vi "STOP.vi"(8 "error in (no error)":errorcluster, 11 "Stop in":refnum<class "DLEmulate.lvclass">) -> (0 "error out":errorcluster, 3 "Stop out":refnum<class "DLEmulate.lvclass">)   [LabVIEW 2015, in "DLEmulate.lvclass"]
uses:
  DLEmulate.lvclass
  GeneralFunctionality/GeneralFunctionality.lvclass/GeneralFunctionality.ctl
  GeneralFunctionality/GeneralFunctionality.lvclass
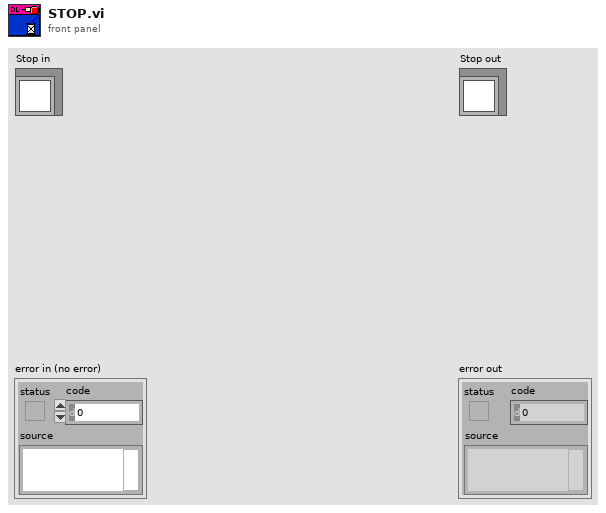
[diagram p1: front panel]
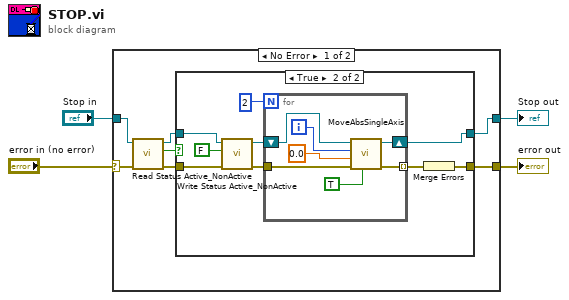
[diagram p0: block diagram]
diagram:
  n1 = case shown="No Error" "error in (no error)" {
    selector: "error in (no error)" -> [w8 w31]
    tunnel: [w11 w31] -> w2
    tunnel: [w5 w30] -> w1
    tunnel: "Stop in" -> [w10 w30]
    frame No Error {
      n2 = call "Read Status Active_NonActive.vi"("error in (no error)"=w8, "GeneralFunctionality in"=w10) -> ("error out"=w7:errorcluster, "Status Active/NonActive"=w6:bool, "GeneralFunctionality out"=w9:refnum<class "DLEmulate.lvclass">)  [unwired: 7 in]
      n3 = case shown="True" w6 {
        tunnel: [w13 w14] -> w11
        tunnel: [w12 w16] -> w5
        tunnel: w9 -> [w12 w21]
        tunnel: w7 -> [w13 w20]
        frame False {
        }
        frame True {
          n4 = call "Write Status Active_NonActive.vi"("error in (no error)"=w20, "Status Active/NonActive"=FALSE, "GeneralFunctionality in"=w21) -> ("error out"=w17:errorcluster, "GeneralFunctionality out"=w19:refnum<class "DLEmulate.lvclass">)  [unwired: 7 in]
          n5 = for {
            N: 2 -> [_]
            tunnel: w17 -> [w26]
            tunnel: [w25] -> w15 mode=indexing
            shift-right: [w24] -> w16
            shift-left: w19 -> [w29]
            i -> [w28]
            n6 = call-dynamic "MoveAbsSingleAxis.vi"("Wait"=TRUE, "error in (no error)"=w26, "Value"=0.0, "Axis"=w28, "DelayLineSimulation in"=w29) -> ("error out"=w25:errorcluster, "DelayLineSimulation out"=w24:refnum<class "DLEmulate.lvclass">)  [unwired: 5 in]
          }
          n7 = Merge Errors(w15) -> (w14:errorcluster)
        }
      }
    }
    frame Error {
    }
  }
  "error out" <- w2
  "Stop out" <- w1
